vi "Get_ACIR_Test_Data.vi"(8 "error in (no error)":errorcluster caption="错误输入（无错误）", 11 "configuration file path":path) -> (0 "error out":errorcluster caption="错误输出", 1 "IR_SET DATA":string[](array[string]), 2 "AC_SET DATA":string[](array[string]))   [LabVIEW 2018]
uses:
  <vilib>/Utility/config.llb/Read Key (String).vi
  Subvi/Global.vi
  <vilib>/Utility/config.llb/NI_LVConfig.lvlib
panel:
  out "OutIRData":string[](array[string])
  out "OutACData":string[](array[string])
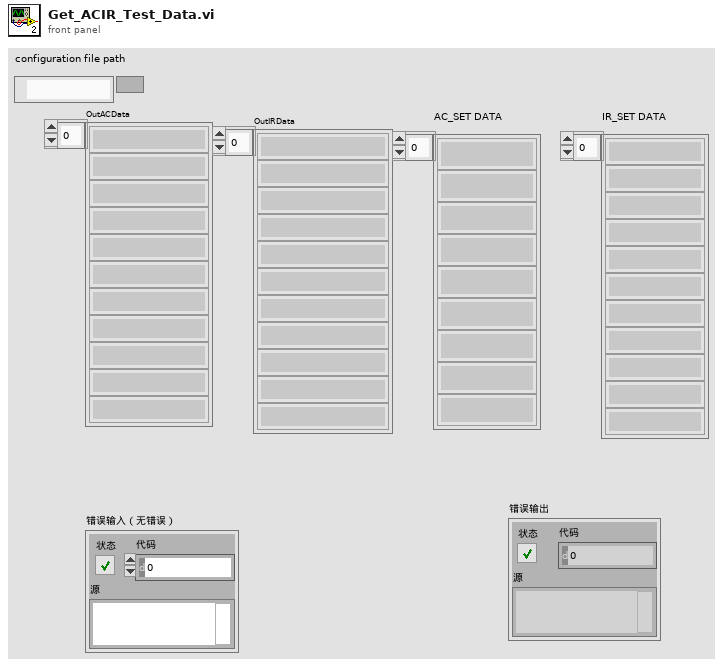
[diagram p1: front panel]
types:
  T1 = typedef "NI_LVConfig.lvlib/Config Data RefNum.ctl" = refnum<k1>
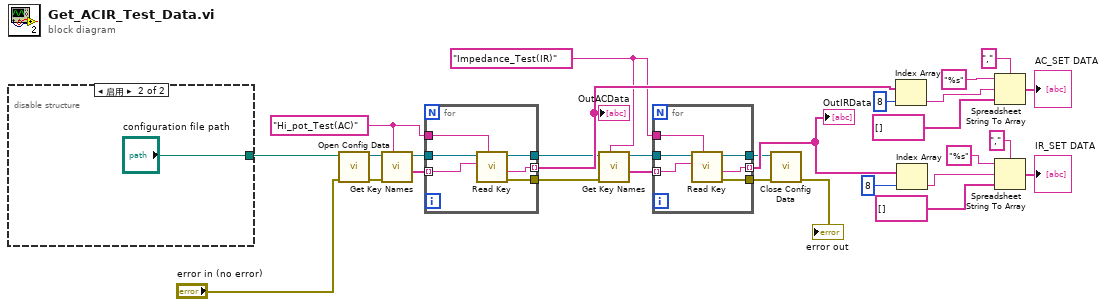
[diagram p0: block diagram]
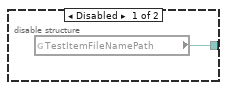
[diagram p2: hidden frame]
diagram:
  w15 = "Impedance_Test(IR)"
  w14 = "Hi_pot_Test(AC)"
  n1 = disable-structure shown="启用" {
    disable-tunnel: [w30 "configuration file path"] -> w29
    frame Disabled {
      n2 = global read "Global.vi" "TestItemFileNamePath"() -> (w30:path)
    }
    frame Enabled {
    }
  }
  n3 = call <vilib>:"Open Config Data.vi"("error in (no error)"="error in (no error)", "configuration file path"=w29) -> ("error out"=w24:errorcluster, "refnum"=w25:T1)  [unwired: 7 in, 1 out]
  n4 = call <vilib>:"Get Key Names.vi"("section"=w14, "error in (no error)"=w24, "refnum"=w25) -> ("key names"=w22:string[], "refnum out"=w23:T1)  [unwired: 5 in, 2 out]
  n5 = for {
    tunnel: w23 -> [w37]
    tunnel: w22 -> [w36] mode=indexing
    tunnel: [w35] -> w28 mode=indexing
    tunnel: w14 -> [w34]
    tunnel: [w33] -> w17
    tunnel: [w32] -> w16
    n6 = call-poly <vilib>:"Read Key.vi"("section"=w34, "key"=w36, "refnum"=w37) -> ("error out"=w32:errorcluster, "value"=w35:string, "refnum out"=w33:T1)  [unwired: 5 in, 1 out]
  }
  "OutACData" <- w28
  n7 = call <vilib>:"Get Key Names.vi"("section"=w15, "error in (no error)"=w16, "refnum"=w17) -> ("key names"=w19:string[], "refnum out"=w18:T1)  [unwired: 5 in, 2 out]
  n8 = for {
    tunnel: w18 -> [w43]
    tunnel: w19 -> [w42] mode=indexing
    tunnel: [w41] -> w27 mode=indexing
    tunnel: w15 -> [w40]
    tunnel: [w39] -> w20
    tunnel: [w38] -> w21
    n9 = call-poly <vilib>:"Read Key.vi"("section"=w40, "key"=w42, "refnum"=w43) -> ("error out"=w38:errorcluster, "value"=w41:string, "refnum out"=w39:T1)  [unwired: 5 in, 1 out]
  }
  "OutIRData" <- w27
  n10 = call <vilib>:"Close Config Data.vi"("error in (no error)"=w21, "refnum"=w20) -> ("error out"=→"error out":errorcluster)  [unwired: 8 in, 1 out]
  n11 = Index Array(array=w28, index=8 ("索引")) -> (element=w13:string)
  n12 = Index Array(array=w27, index=8 ("索引")) -> (element=w10:string)
  n13 = Spreadsheet String To Array(delimiter (Tab)="," ("分隔符(Tab)"), format string="%s" ("格式字符串"), spreadsheet string=w13, array type (2D Dbl)=string[] []) -> (array=→"AC_SET DATA":string[])
  n14 = Spreadsheet String To Array(delimiter (Tab)="," ("分隔符(Tab)"), format string="%s" ("格式字符串"), spreadsheet string=w10, array type (2D Dbl)=string[] []) -> (array=→"IR_SET DATA":string[])
